vi "PCO_ConvertGet.vi"(8 "error in (no error)":errorcluster {"code" format="%x"}, 11 "ph":u64) -> (0 "error out":errorcluster {"code" format="%x"}, 1 "strConvert":T1, 2 "ErrorMessage":i32 format="%x", 3 "ph out":u64)   [LabVIEW 2019, in "Convert.lvlib"]
doc: "int PCOCONVERT_API PCO_ConvertGet(HANDLE ph, PCO_Convert* pstrConvert);"
uses:
  Convert.lvlib
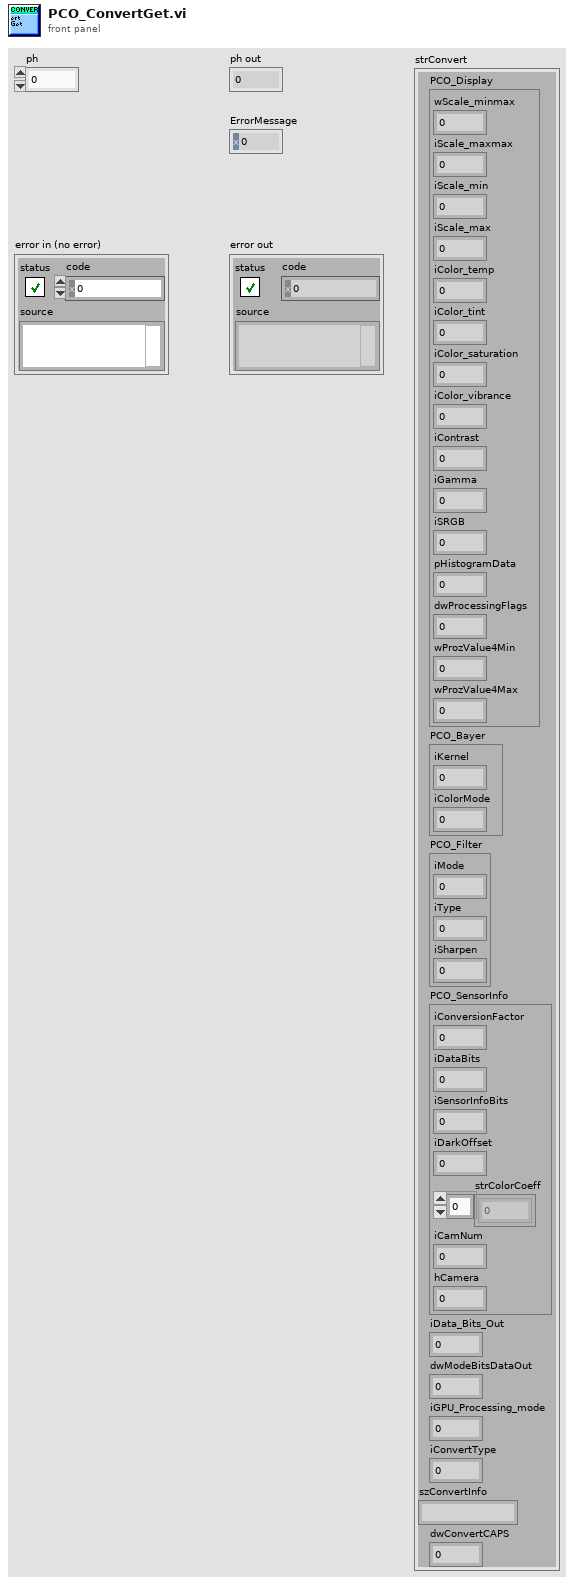
[diagram p1: front panel]
types:
  T1 = cluster{"PCO_Display":cluster{"wScale_minmax":u16, "iScale_maxmax":i32, "iScale_min":i32, "iScale_max":i32, "iColor_temp":i32, "iColor_tint":i32, "iColor_saturation":i32, "iColor_vibrance":i32, "iContrast":i32, "iGamma":i32, "iSRGB":i32, "pHistogramData":u64, "dwProcessingFlags":u32, "wProzValue4Min":u16, "wProzValue4Max":u16}, "PCO_Bayer":cluster{"iKernel":i32, "iColorMode":i32}, "PCO_Filter":cluster{"iMode":i32, "iType":i32, "iSharpen":i32}, "PCO_SensorInfo":cluster{"iConversionFactor":i32, "iDataBits":i32, "iSensorInfoBits":i32, "iDarkOffset":i32, "strColorCoeff":dbl[], "iCamNum":i32, "hCamera":u64}, "iData_Bits_Out":i32, "dwModeBitsDataOut":u32, "iGPU_Processing_mode":i32, "iConvertType":i32, "szConvertInfo":string, "dwConvertCAPS":u32}
  T2 = cluster{"wSize":u16, "wDummy":cluster{u16, u16, u16}, "PCO_DisplayRaw_x64":cluster{"wSize":u16, "wScale_minmax":u16, "iScale_maxmax":i32, "iScale_min":i32, "iScale_max":i32, "iColor_temp":i32, "iColor_tint":i32, "iColor_saturation":i32, "iColor_vibrance":i32, "iContrast":i32, "iGamma":i32, "iSRGB":i32, "pHistogramData":u64, "dwDialogOpenFlags":u32, "dwProcessingFlags":u32, "wProzValue4Min":u16, "wProzValue4Max":u16, "dwzzDummy1":cluster{u32, u32, u32, u32, u32, u32, u32, u32, u32, u32, u32, u32, u32, u32, u32, u32, u32, u32, u32, u32, u32, u32, u32, u32, u32, u32, u32, u32, u32, u32, u32, u32, u32, u32, u32, u32, u32, u32, u32, u32, u32, u32, u32, u32, u32, u32, u32, u32, u32, u32}}, "PCO_Bayer_Raw":cluster{"wSize":u16, "wDummy":u16, "iKernel":i32, "iColorMode":i32, "dwzzDummy1":cluster{u32, u32, u32, u32, u32, u32, u32, u32, u32, u32, u32, u32, u32, u32, u32, u32, u32, u32, u32, u32, u32, u32, u32, u32, u32, u32, u32, u32, u32, u32, u32, u32, u32, u32, u32, u32, u32, u32, u32, u32, u32, u32, u32, u32, u32, u32, u32, u32, u32, u32, u32, u32, u32, u32, u32, u32, u32, u32, u32, u32, u32}}, "PCO_Filter_Raw":cluster{"wSize":u16, "wDummy":u16, "iMode":i32, "iType":i32, "iSharpen":i32, "dwzzDummy1":cluster{u32, u32, u32, u32, u32, u32, u32, u32, u32, u32, u32, u32, u32, u32, u32, u32, u32, u32, u32, u32, u32, u32, u32, u32, u32, u32, u32, u32, u32, u32, u32, u32, u32, u32, u32, u32, u32, u32, u32, u32, u32, u32, u32, u32, u32, u32, u32, u32, u32, u32, u32, u32, u32, u32, u32, u32, u32, u32, u32, u32}}, "PCO_SensorInfo_Raw_x64":cluster{"wSize":u16, "wDummy":u16, "iConversionFactor":i32, "iDataBits":i32, "iSensorInfoBits":i32, "iDarkOffset":i32, "dwzzDummy0":u32, "strColorCoeff":cluster{dbl, dbl, dbl, dbl, dbl, dbl, dbl, dbl, dbl}, "iCamNum":i32, "hCamera":u64, "dwzzDummy1":cluster{u32, u32, u32, u32, u32, u32, u32, u32, u32, u32, u32, u32, u32, u32, u32, u32, u32, u32, u32, u32, u32, u32, u32, u32, u32, u32, u32, u32, u32, u32, u32, u32, u32, u32, u32, u32, u32, u32, u32}}, "iData_Bits_Out":i32, "dwModeBitsDataOut":u32, "iGPU_Processing_mode":i32, "iConvertType":i32, "szConvertInfo":cluster{u8, u8, u8, u8, u8, u8, u8, u8, u8, u8, u8, u8, u8, u8, u8, u8, u8, u8, u8, u8, u8, u8, u8, u8, u8, u8, u8, u8, u8, u8, u8, u8, u8, u8, u8, u8, u8, u8, u8, u8, u8, u8, u8, u8, u8, u8, u8, u8, u8, u8, u8, u8, u8, u8, u8, u8, u8, u8, u8, u8}, "dwConvertCAPS":u32, "dwzzDummy1":cluster{u32, u32, u32, u32, u32, u32, u32, u32, u32, u32, u32, u32, u32, u32, u32, u32, u32, u32, u32, u32, u32, u32, u32, u32, u32, u32, u32, u32, u32, u32, u32, u32, u32, u32, u32, u32, u32, u32, u32, u32, u32, u32}}
  T3 = cluster{"wSize":u16, "wDummy":cluster{u16, u16, u16}, "PCO_DisplayRaw_win32":cluster{"wSize":u16, "wScale_minmax":u16, "iScale_maxmax":i32, "iScale_min":i32, "iScale_max":i32, "iColor_temp":i32, "iColor_tint":i32, "iColor_saturation":i32, "iColor_vibrance":i32, "iContrast":i32, "iGamma":i32, "iSRGB":i32, "pHistogramData":u32, "dwDialogOpenFlags":u32, "dwProcessingFlags":u32, "wProzValue4Min":u16, "wProzValue4Max":u16, "dwzzDummy1":cluster{u32, u32, u32, u32, u32, u32, u32, u32, u32, u32, u32, u32, u32, u32, u32, u32, u32, u32, u32, u32, u32, u32, u32, u32, u32, u32, u32, u32, u32, u32, u32, u32, u32, u32, u32, u32, u32, u32, u32, u32, u32, u32, u32, u32, u32, u32, u32, u32, u32}}, "PCO_Bayer_Raw":cluster{"wSize":u16, "wDummy":u16, "iKernel":i32, "iColorMode":i32, "dwzzDummy1":cluster{u32, u32, u32, u32, u32, u32, u32, u32, u32, u32, u32, u32, u32, u32, u32, u32, u32, u32, u32, u32, u32, u32, u32, u32, u32, u32, u32, u32, u32, u32, u32, u32, u32, u32, u32, u32, u32, u32, u32, u32, u32, u32, u32, u32, u32, u32, u32, u32, u32, u32, u32, u32, u32, u32, u32, u32, u32, u32, u32, u32, u32}}, "PCO_Filter_Raw":cluster{"wSize":u16, "wDummy":u16, "iMode":i32, "iType":i32, "iSharpen":i32, "dwzzDummy1":cluster{u32, u32, u32, u32, u32, u32, u32, u32, u32, u32, u32, u32, u32, u32, u32, u32, u32, u32, u32, u32, u32, u32, u32, u32, u32, u32, u32, u32, u32, u32, u32, u32, u32, u32, u32, u32, u32, u32, u32, u32, u32, u32, u32, u32, u32, u32, u32, u32, u32, u32, u32, u32, u32, u32, u32, u32, u32, u32, u32, u32}}, "PCO_SensorInfo_Raw_win32":cluster{"wSize":u16, "wDummy":u16, "iConversionFactor":i32, "iDataBits":i32, "iSensorInfoBits":i32, "iDarkOffset":i32, "dwzzDummy0":u32, "strColorCoeff":cluster{dbl, dbl, dbl, dbl, dbl, dbl, dbl, dbl, dbl}, "iCamNum":i32, "hCamera":u32, "dwzzDummy1":cluster{u32, u32, u32, u32, u32, u32, u32, u32, u32, u32, u32, u32, u32, u32, u32, u32, u32, u32, u32, u32, u32, u32, u32, u32, u32, u32, u32, u32, u32, u32, u32, u32, u32, u32, u32, u32, u32, u32}}, "iData_Bits_Out":i32, "dwModeBitsDataOut":u32, "iGPU_Processing_mode":i32, "iConvertType":i32, "szConvertInfo":cluster{u8, u8, u8, u8, u8, u8, u8, u8, u8, u8, u8, u8, u8, u8, u8, u8, u8, u8, u8, u8, u8, u8, u8, u8, u8, u8, u8, u8, u8, u8, u8, u8, u8, u8, u8, u8, u8, u8, u8, u8, u8, u8, u8, u8, u8, u8, u8, u8, u8, u8, u8, u8, u8, u8, u8, u8, u8, u8, u8, u8}, "dwConvertCAPS":u32, "dwzzDummy1":cluster{u32, u32, u32, u32, u32, u32, u32, u32, u32, u32, u32, u32, u32, u32, u32, u32, u32, u32, u32, u32, u32, u32, u32, u32, u32, u32, u32, u32, u32, u32, u32, u32, u32, u32, u32, u32, u32, u32, u32, u32, u32, u32}}
  T4 = cluster{"wSize":u16, "wScale_minmax":u16, "iScale_maxmax":i32, "iScale_min":i32, "iScale_max":i32, "iColor_temp":i32, "iColor_tint":i32, "iColor_saturation":i32, "iColor_vibrance":i32, "iContrast":i32, "iGamma":i32, "iSRGB":i32, "pHistogramData":u64, "dwDialogOpenFlags":u32, "dwProcessingFlags":u32, "wProzValue4Min":u16, "wProzValue4Max":u16, "dwzzDummy1":cluster{u32, u32, u32, u32, u32, u32, u32, u32, u32, u32, u32, u32, u32, u32, u32, u32, u32, u32, u32, u32, u32, u32, u32, u32, u32, u32, u32, u32, u32, u32, u32, u32, u32, u32, u32, u32, u32, u32, u32, u32, u32, u32, u32, u32, u32, u32, u32, u32, u32, u32}}
  T5 = cluster{"wSize":u16, "wDummy":u16, "iKernel":i32, "iColorMode":i32, "dwzzDummy1":cluster{u32, u32, u32, u32, u32, u32, u32, u32, u32, u32, u32, u32, u32, u32, u32, u32, u32, u32, u32, u32, u32, u32, u32, u32, u32, u32, u32, u32, u32, u32, u32, u32, u32, u32, u32, u32, u32, u32, u32, u32, u32, u32, u32, u32, u32, u32, u32, u32, u32, u32, u32, u32, u32, u32, u32, u32, u32, u32, u32, u32, u32}}
  T6 = cluster{"wSize":u16, "wDummy":u16, "iMode":i32, "iType":i32, "iSharpen":i32, "dwzzDummy1":cluster{u32, u32, u32, u32, u32, u32, u32, u32, u32, u32, u32, u32, u32, u32, u32, u32, u32, u32, u32, u32, u32, u32, u32, u32, u32, u32, u32, u32, u32, u32, u32, u32, u32, u32, u32, u32, u32, u32, u32, u32, u32, u32, u32, u32, u32, u32, u32, u32, u32, u32, u32, u32, u32, u32, u32, u32, u32, u32, u32, u32}}
  T7 = cluster{"wSize":u16, "wDummy":u16, "iConversionFactor":i32, "iDataBits":i32, "iSensorInfoBits":i32, "iDarkOffset":i32, "dwzzDummy0":u32, "strColorCoeff":cluster{dbl, dbl, dbl, dbl, dbl, dbl, dbl, dbl, dbl}, "iCamNum":i32, "hCamera":u64, "dwzzDummy1":cluster{u32, u32, u32, u32, u32, u32, u32, u32, u32, u32, u32, u32, u32, u32, u32, u32, u32, u32, u32, u32, u32, u32, u32, u32, u32, u32, u32, u32, u32, u32, u32, u32, u32, u32, u32, u32, u32, u32, u32}}
  T8 = cluster{u8, u8, u8, u8, u8, u8, u8, u8, u8, u8, u8, u8, u8, u8, u8, u8, u8, u8, u8, u8, u8, u8, u8, u8, u8, u8, u8, u8, u8, u8, u8, u8, u8, u8, u8, u8, u8, u8, u8, u8, u8, u8, u8, u8, u8, u8, u8, u8, u8, u8, u8, u8, u8, u8, u8, u8, u8, u8, u8, u8}
  T9 = cluster{dbl, dbl, dbl, dbl, dbl, dbl, dbl, dbl, dbl}
  T10 = cluster{"iConversionFactor":i32, "iDataBits":i32, "iSensorInfoBits":i32, "iDarkOffset":i32, "strColorCoeff":dbl[], "iCamNum":i32, "hCamera":u64}
  T11 = cluster{"iMode":i32, "iType":i32, "iSharpen":i32}
  T12 = cluster{"wScale_minmax":u16, "iScale_maxmax":i32, "iScale_min":i32, "iScale_max":i32, "iColor_temp":i32, "iColor_tint":i32, "iColor_saturation":i32, "iColor_vibrance":i32, "iContrast":i32, "iGamma":i32, "iSRGB":i32, "pHistogramData":u64, "dwProcessingFlags":u32, "wProzValue4Min":u16, "wProzValue4Max":u16}
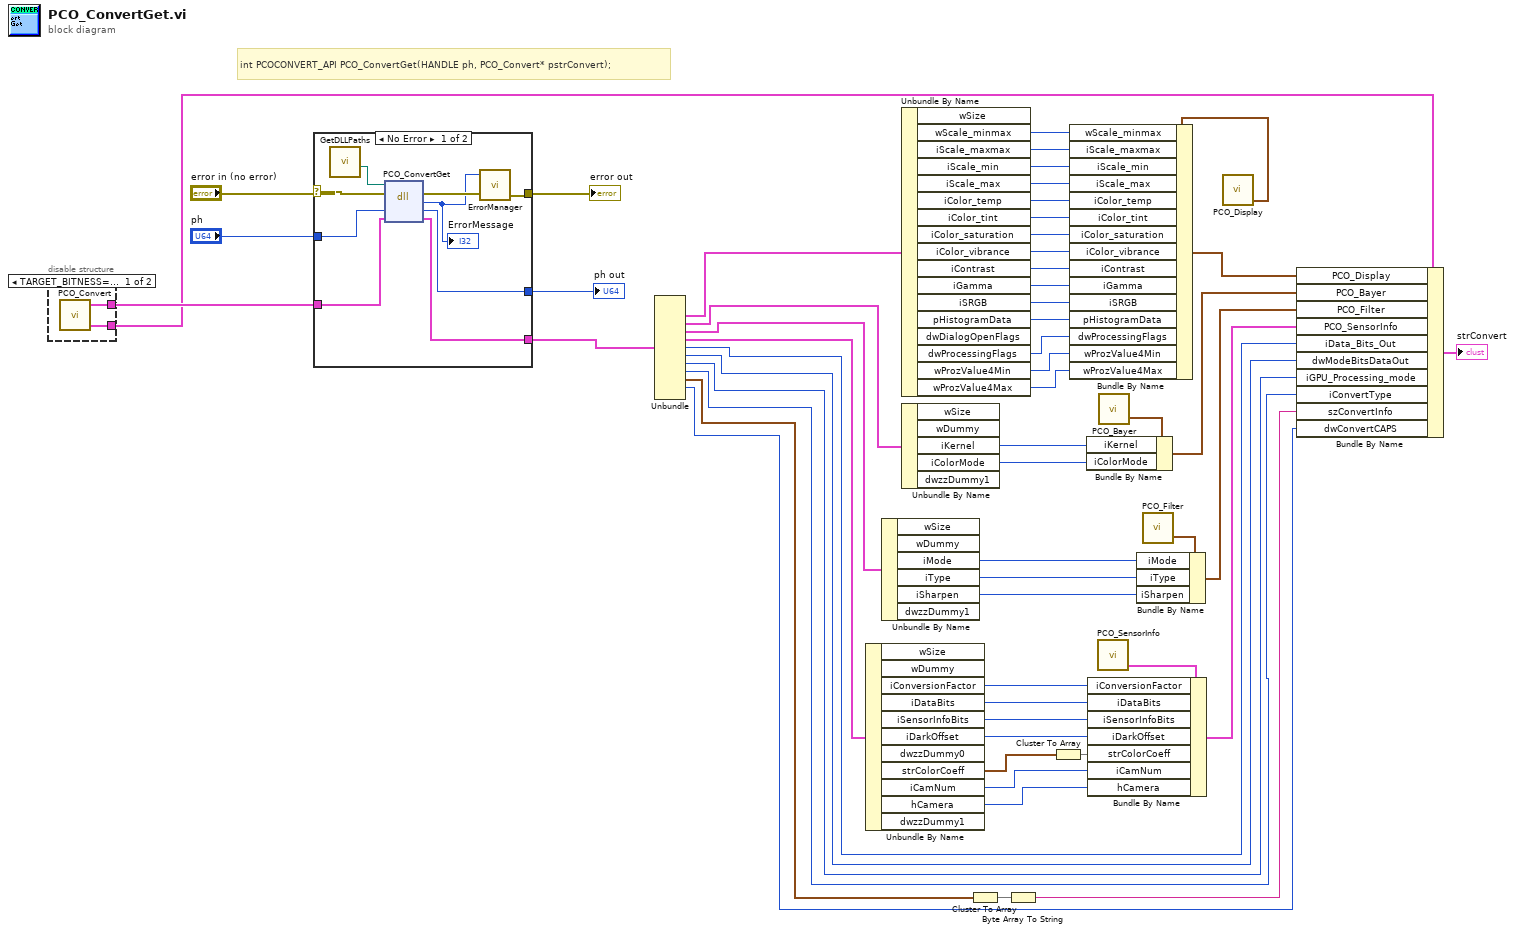
[diagram p0: block diagram]
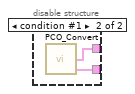
[diagram p2: hidden frame]
diagram:
  # "int PCOCONVERT_API PCO_ConvertGet(HANDLE ph, PCO_Convert* pstrConvert);"
  n1 = disable-structure "Diagram Disable Structure" shown="TARGET_BITNESS==64, Default" {
    disable-tunnel: [w58 w60] -> w51
    disable-tunnel: [w57 w59] -> w52
    frame condition #0 (active) {
      n2 = call "PCO_Convert.vi"() -> ("PCO_ConvertRaw_x64"=w57:T2, "PCO_Convert"=w58:T1)  [unwired: 4 in, 3 out]
    }
    frame condition #1 {
      n3 = call "PCO_Convert.vi"() -> ("PCO_ConvertRaw_win32"=w59:T3, "PCO_Convert"=w60:T1)  [unwired: 4 in, 3 out]
    }
  }
  n4 = case shown="No Error" "error in (no error)" {
    selector: "error in (no error)" -> [w65 w70]
    tunnel: "ph" -> [w69 w72]
    tunnel: [w68 w72] -> w55
    tunnel: w52 -> [w67 w71]
    tunnel: [w66 w71] -> w17
    tunnel: [w63 w70] -> w54
    frame No Error {
      n5 = call "GetDLLPaths.vi"() -> ("PCO_Conv_Path"=w61:path)  [unwired: 9 in, 2 out]
      n6 = dll-call lib="?" fn="PCO_ConvertGet"(path in=w61, error in=w65, "ph"=w69, "pstrConvert"=w67) -> (error out=w64:errorcluster, "return type"=w62:i32, "ph"=w68:u64, "pstrConvert"=w66:T2)  [unwired: 1 in, 1 out]
      "ErrorMessage" <- w62
      n7 = call "ErrorManager.vi"("error in (no error)"=w64, "error code"=w62) -> ("error out"=w63:errorcluster)  [unwired: 3 in]
    }
    frame Error {
    }
  }
  "ph out" <- w55
  "error out" <- w54
  n8 = Unbundle(w17) -> ("PCO_DisplayRaw_x64"=w16:T4, "PCO_Bayer_Raw"=w15:T5, "PCO_Filter_Raw"=w14:T6, "PCO_SensorInfo_Raw_x64"=w13:T7, "iData_Bits_Out"=w12:i32, "dwModeBitsDataOut"=w11:u32, "iGPU_Processing_mode"=w10:i32, "iConvertType"=w9:i32, "szConvertInfo"=w4:T8, "dwConvertCAPS"=w1:u32)  [unwired: 3 out]
  n9 = Unbundle By Name(w13) -> ("iConversionFactor"=w49:i32, "iDataBits"=w48:i32, "iSensorInfoBits"=w47:i32, "iDarkOffset"=w46:i32, "strColorCoeff"=w45:T9, "iCamNum"=w43:i32, "hCamera"=w42:u64)  [unwired: 4 out]
  n10 = Unbundle By Name(w14) -> ("iMode"=w37:i32, "iType"=w38:i32, "iSharpen"=w39:i32)  [unwired: 3 out]
  n11 = Unbundle By Name(w16) -> ("wScale_minmax"=w29:u16, "iScale_maxmax"=w28:i32, "iScale_min"=w27:i32, "iScale_max"=w26:i32, "iColor_temp"=w25:i32, "iColor_tint"=w24:i32, "iColor_saturation"=w23:i32, "iColor_vibrance"=w22:i32, "iContrast"=w21:i32, "iGamma"=w20:i32, "iSRGB"=w19:i32, "pHistogramData"=w18:u64, "dwProcessingFlags"=w8:u32, "wProzValue4Min"=w7:u16, "wProzValue4Max"=w6:u16)  [unwired: 2 out]
  n12 = Unbundle By Name(w15) -> ("iKernel"=w34:i32, "iColorMode"=w33:i32)  [unwired: 3 out]
  n13 = Cluster To Array(cluster=w4) -> (array=w3:u8[])
  n14 = Byte Array To String(unsigned byte array=w3) -> (string=w2:string)
  n15 = Cluster To Array(cluster=w45) -> (array=w44:dbl[])
  n16 = call "PCO_SensorInfo.vi"() -> ("PCO_SensorInfo"=w50:T10)  [unwired: 4 in, 4 out]
  n17 = Bundle By Name(cluster=w50, "iConversionFactor"=w49, "iDataBits"=w48, "iSensorInfoBits"=w47, "iDarkOffset"=w46, "strColorCoeff"=w44, "iCamNum"=w43, "hCamera"=w42) -> (w41:T10)
  n18 = call "PCO_Bayer.vi"() -> ("PCO_Bayer"=w35:cluster{"iKernel":i32, "iColorMode":i32})  [unwired: 4 in, 3 out]
  n19 = Bundle By Name(cluster=w35, "iKernel"=w34, "iColorMode"=w33) -> (w32:cluster{"iKernel":i32, "iColorMode":i32})
  n20 = call "PCO_Filter.vi"() -> ("PCO_Filter"=w40:T11)  [unwired: 4 in, 3 out]
  n21 = Bundle By Name(cluster=w40, "iMode"=w37, "iType"=w38, "iSharpen"=w39) -> (w36:T11)
  n22 = call "PCO_Display.vi"() -> ("PCO_Display"=w31:T12)  [unwired: 4 in, 4 out]
  n23 = Bundle By Name(cluster=w31, "wScale_minmax"=w29, "iScale_maxmax"=w28, "iScale_min"=w27, "iScale_max"=w26, "iColor_temp"=w25, "iColor_tint"=w24, "iColor_saturation"=w23, "iColor_vibrance"=w22, "iContrast"=w21, "iGamma"=w20, "iSRGB"=w19, "pHistogramData"=w18, "dwProcessingFlags"=w8, "wProzValue4Min"=w7, "wProzValue4Max"=w6) -> (w30:T12)
  n24 = Bundle By Name(cluster=w51, "PCO_Display"=w30, "PCO_Bayer"=w32, "PCO_Filter"=w36, "PCO_SensorInfo"=w41, "iData_Bits_Out"=w12, "dwModeBitsDataOut"=w11, "iGPU_Processing_mode"=w10, "iConvertType"=w9, "szConvertInfo"=w2, "dwConvertCAPS"=w1) -> (→"strConvert":T1)
